vi "GET-SET_POWER_ENABLE_1.0.0.vi"(4 "Timeout":u32=3000, 5 "Delay Time (ms)":dbl=1.0 caption="Delay Time (s)", 6 "Get Power Only (T)":bool, 7 "Pwr ON SET (T)":bool, 8 "error in":errorcluster {"code" format="%.0x"}, 11 "Session In":refnum<visa-resource-name>="GPIB0::22::INSTR") -> (0 "error out":errorcluster {"code" format="%.0x"}, 2 "Get Power":dbl, 3 "Session Out":refnum<visa-resource-name>)   [LabVIEW 2018]
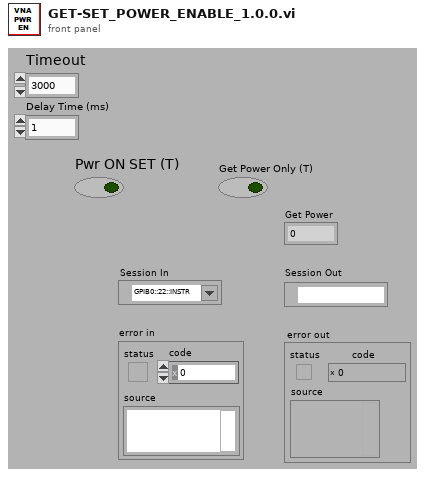
[diagram p1: front panel]
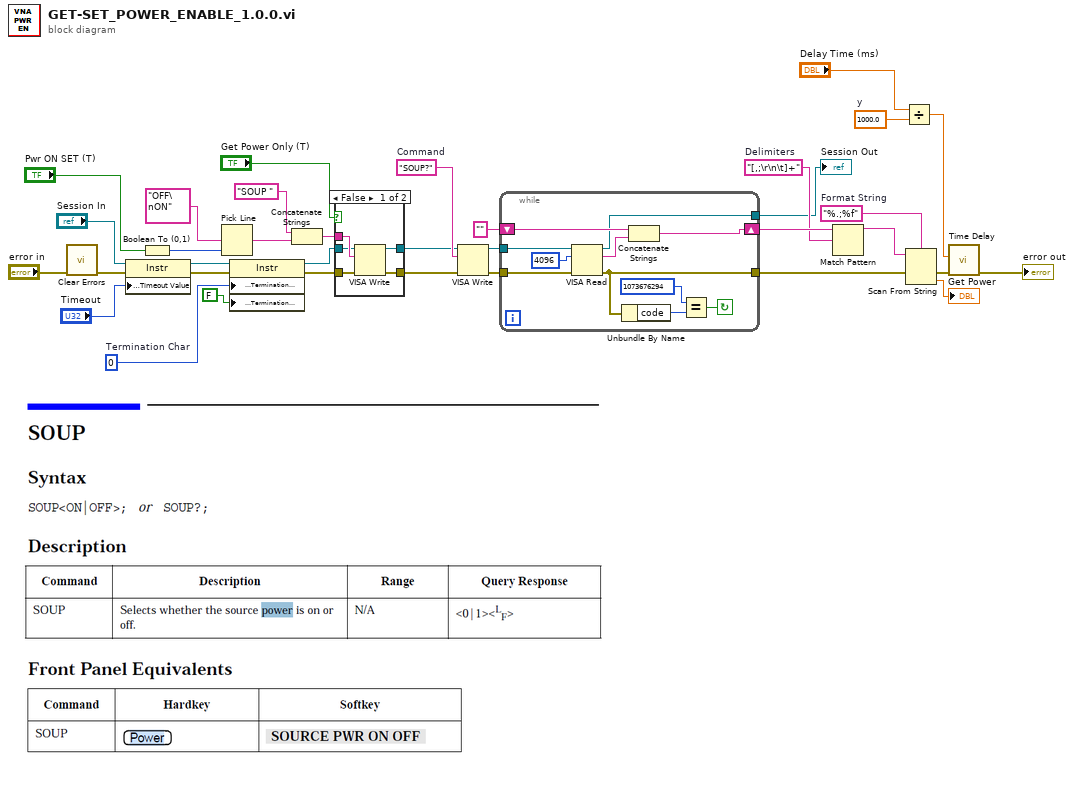
[diagram p0: block diagram]
diagram:
  w1 = 1000.0  # y
  w15 = "[,;\r\n\t]+"  # Delimiters
  w17 = "%.;%f"  # Format String
  w20 = "SOUP?"  # Command
  w30 = u8 0  # Termination Char
  n1 = call <vilib>:"Clear Errors.vi"("error in (no error)"="error in") -> ("error out"=w12:errorcluster)  [unwired: 5 in, 1 out]
  n2 = property class="Instr"(reference="Session In", error in=w12, "General Settings:Timeout Value"="Timeout") -> (reference out=w29:refnum<visa-resource-name>, error out=w32:errorcluster)
  n3 = Boolean To (0,1)(Boolean="Pwr ON SET (T)") -> (0, 1=w7:i16)
  n4 = Pick Line(multi-line string="OFF\nON", line index=w7) -> (output string=w6:string)  [unwired: 1 in]
  n5 = property class="Instr"(reference=w29, error in=w32, "Message Based Settings:Termination Character"=w30, "Message Based Settings:Termination Character Enable"=FALSE ("enable")) -> (reference out=w14:refnum<visa-resource-name>, error out=w31:errorcluster)
  n6 = Concatenate Strings("SOUP " ("staticText"), w6) -> (w25:string)
  n7 = case shown="False" "Get Power Only (T)" {
    tunnel: w31 -> [w40 w42]
    tunnel: [w39 w42] -> w26
    tunnel: w25 -> [w38 _]
    tunnel: w14 -> [w37 w41]
    tunnel: [w36 w41] -> w9
    frame False {
      n8 = VISA Write(VISA resource name=w37, write buffer=w38, error in (no error)=w40) -> (VISA resource name out=w36:refnum<visa-resource-name>, error out=w39:errorcluster)  [unwired: 1 out]
    }
    frame True {
    }
  }
  n9 = VISA Write(VISA resource name=w9, write buffer=w20, error in (no error)=w26) -> (VISA resource name out=w24:refnum<visa-resource-name>, error out=w23:errorcluster)  [unwired: 1 out]
  n10 = while {
    tunnel: w24 -> [w50]
    shift-right: [w44] -> w19
    shift-left: "" -> [w49]
    tunnel: w23 -> [w47]
    tunnel: [w46] -> w22
    tunnel: [w43] -> w11
    stop <- w45 continue-if-true
    n11 = VISA Read(VISA resource name=w50, byte count=u32 4096 ("byte count (0)"), error in (no error)=w47) -> (VISA resource name out=w43:refnum<visa-resource-name>, read buffer=w48:string, error out=w46:errorcluster)  [unwired: 1 out]
    n12 = Unbundle By Name(w46) -> ("code"=w52:i32)
    n13 = Concatenate Strings(w49, w48) -> (w44:string)
    n14 = Equal?(x=1073676294, y=w52) -> (x = y?=w45:bool)
  }
  "Session Out" <- w11
  n15 = Match Pattern(string=w19, regular expression=w15) -> (before substring=w18:string)  [unwired: 1 in, 3 out]
  n16 = Divide(x="Delay Time (ms)", y=w1) -> (x/y=w3:dbl)
  n17 = Scan From String(format string=w17, input string=w18, error in=w22) -> (error out=w4:errorcluster, output 1=→"Get Power":dbl)  [unwired: 2 in, 2 out]
  n18 = call "Time Delay"("error in (no error)"=w4, "Delay Time (s)"=w3) -> ("error out"=→"error out":errorcluster)  [unwired: 9 in]
